vi "TestDevicesList.vi"() -> (1 "Names":string[](array[string]), 2 "Array":T1[](array[typedef]))   [LabVIEW 2017]
uses:
  <vilib>/addons/InsightCM/MessageBus/MessageLibrary/SysCfgDeployer/controls/SysCfgDeployPackageRequestBody.ctl
  <vilib>/Utility/file.llb/Read Delimited Spreadsheet (string).vi
panel:
  out "all rows":string[][](array[string])
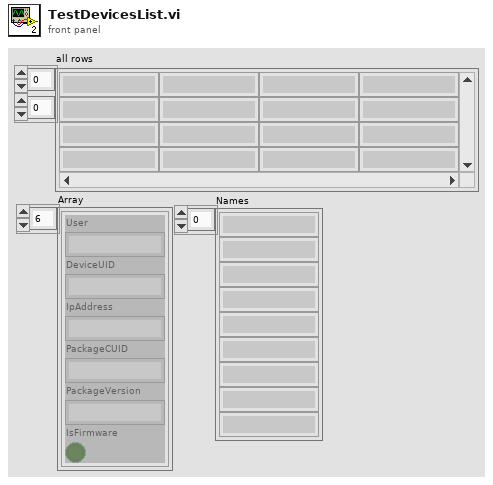
[diagram p1: front panel]
types:
  T1 = typedef "SysCfgDeployPackageRequestBody.ctl" = cluster{"User":string, "DeviceUID":string, "IpAddress":string, "PackageCUID":string, "PackageVersion":string, "IsFirmware":bool}
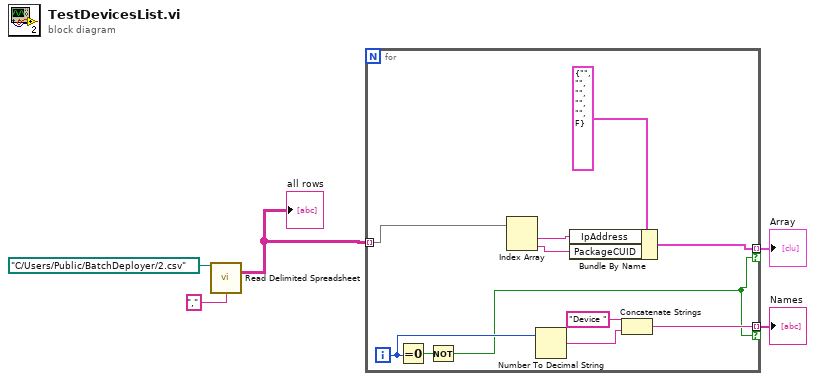
[diagram p0: block diagram]
diagram:
  n1 = call-poly <vilib>:"Read Delimited Spreadsheet.vi"("file path (dialog if empty)"=path "C:/Users/Public/BatchDeployer/2.csv", "delimiter (\\t)"="," ("delimiter (\\t)")) -> ("all rows"=w3:string[][])  [unwired: 8 in, 5 out]
  "all rows" <- w3
  n2 = for {
    tunnel: w3 -> [w16] mode=indexing
    tunnel: [w15] -> w2 mode=indexing if=w6
    tunnel: [w7] -> w1 mode=indexing if=w6
    i -> [w8]
    n3 = Equal To 0?(x=w8) -> (x = 0?=w14:bool)
    n4 = Not(x=w14) -> (.not. x?=w6:bool)
    n5 = Index Array(array=w16) -> (element #1=w12:string, element #2=w11:string)  [unwired: 2 in]
    n6 = Number To Decimal String(number=w8) -> (decimal integer string=w9:string)  [unwired: 1 in]
    n7 = Bundle By Name(cluster=T1 {"User"="", "DeviceUID"="", "IpAddress"="", "PackageCUID"="", "PackageVersion"="", "IsFirmware"=FALSE} ("SysCfgDeployRequest"), "IpAddress"=w12, "PackageCUID"=w11) -> (w15:T1)
    n8 = Concatenate Strings("Device ", w9) -> (w7:string)
  }
  "Array" <- w2
  "Names" <- w1
